vi "Write Conflicts to Table.vi"(8 "error in (no error)":errorcluster, 10 "Conflicts":T1(array[cluster]), 11 "MC Listbox Ref":refnum<vi>) -> (0 "error out":errorcluster)   [LabVIEW 2020, in "Modbus Master System Explorer.lvlib"]
uses:
  Modbus Master System Explorer.lvlib
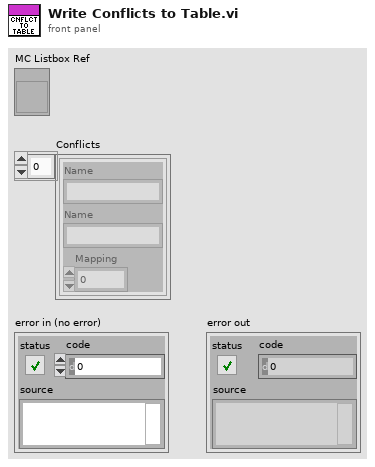
[diagram p1: front panel]
types:
  T1 = cluster{"Name":string, "Name":string, "Mapping":u16}[]
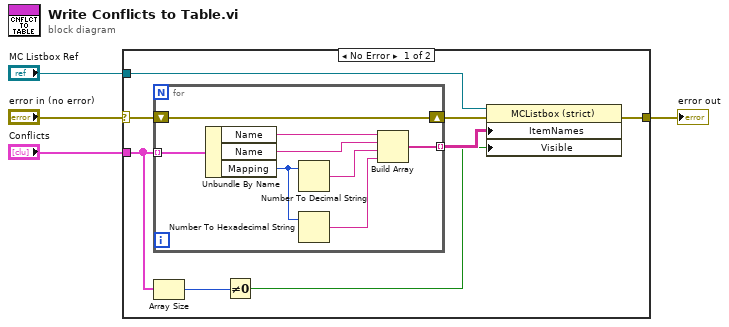
[diagram p0: block diagram]
diagram:
  n1 = case shown="No Error" "error in (no error)" {
    selector: "error in (no error)" -> [w7 w21]
    tunnel: "MC Listbox Ref" -> [w12 _]
    tunnel: "Conflicts" -> [w10 _]
    tunnel: [w5 w21] -> w1
    frame No Error {
      n2 = for {
        tunnel: w10 -> [w20] mode=indexing
        tunnel: [w17] -> w11 mode=indexing
        shift-right: [w16] -> w6
        shift-left: w7 -> [w16]
        n3 = Unbundle By Name(w20) -> ("Name"=w19:string, "Name"=w18:string, "Mapping"=w14:u16)
        n4 = Number To Decimal String(number=w14) -> (decimal integer string=w15:string)  [unwired: 1 in]
        n5 = Number To Hexadecimal String(2:w14) -> (0:w13:string)  [unwired: 1 in]
        n6 = Build Array(w19, w18, w15, w13) -> (w17:string[])
      }
      n7 = Array Size(array=w10) -> (size(s)=w9:i32)
      n8 = Not Equal To 0?(x=w9) -> (x != 0?=w8:bool)
      n9 = property on="Property Node" class="MCListbox (strict)"(reference=w12, error in=w6, "ItemNames"=w11, "Visible"=w8) -> (error out=w5:errorcluster)  [unwired: 1 out]
    }
    frame Error {
    }
  }
  "error out" <- w1
